vi "sendFixedData.vi"(8 "error in (no error)":errorcluster, 9 "File name wo extension":string="AdminConfig", 10 "File contents":string, 11 "SM1000-control in":T1) -> (0 "error out":errorcluster, 3 "SM1000-control out":T1)   [LabVIEW 2013, in "SLMControl.lvlib" / "SM1000.lvclass"]
doc: "Send fixed data to an EC device session.\n\nData retrieved via the 'requestFixedData' method may be modified and passed back to the controller for local storage. That data will then be immediately used and also the next time the module is booted.\nAn application should wait on an application message event 'FixedDataProcessed' to be assured the updated data has been processed by the EC1000 and is ready for subsequent actions."
uses:
  SM1000.lvclass
  Object-reference.ctl
  SM1000.lvclass/SM1000.ctl
  Custom-errors.ctl
  C:/Users/vangeste/Desktop/2015-06-02 - SLM - MAIF/HC-HardwareCharacterization/Sources/SM1000/LECSession.dll
  HC-HardwareCharacterization/Sources/SM1000/LECSession.dll
  DOTNET-error-int.vi
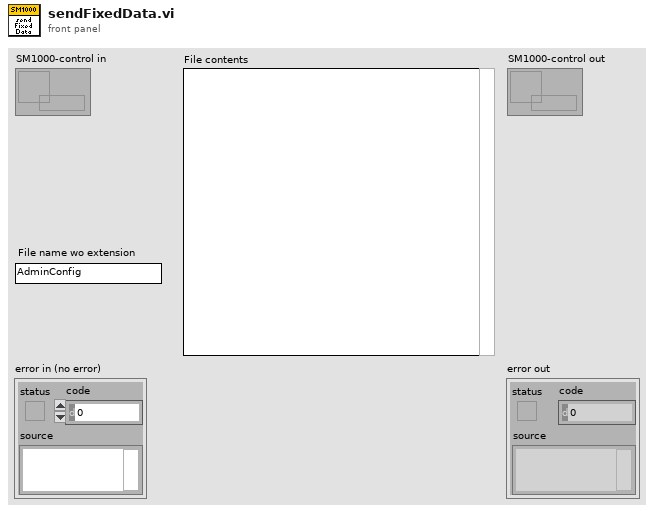
[diagram p1: front panel]
types:
  T1 = typedef "SLMControl.lvlib/SM1000.lvclass/Object-reference.ctl" = refnum<data-value>
  T2 = typedef "SLMControl.lvlib/SM1000.lvclass/Custom-errors.ctl" = enum16{"No error", "Not implemented", "Command not recognized", "Invalid input", "No connection", "Timeout", "Resource not loaded"}
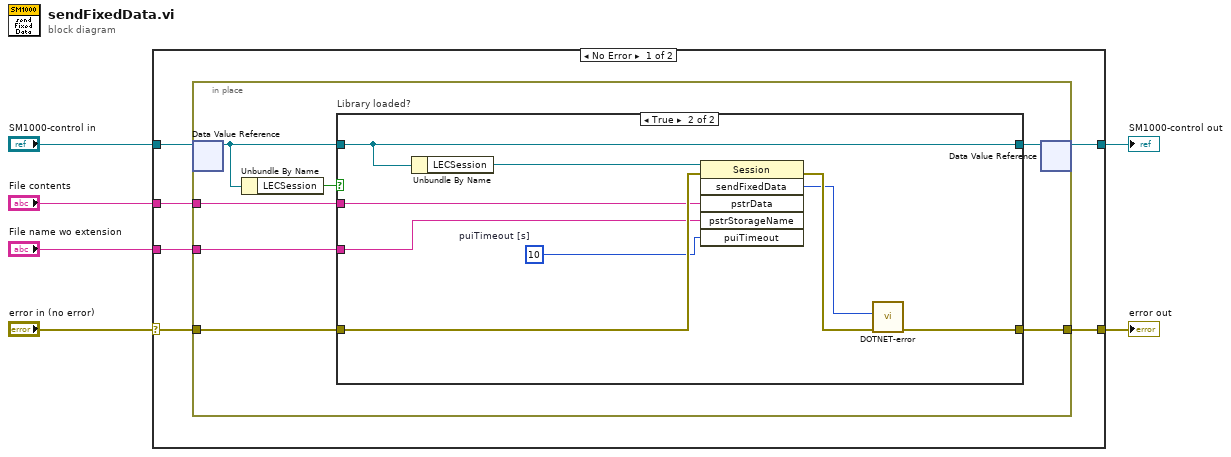
[diagram p0: block diagram]
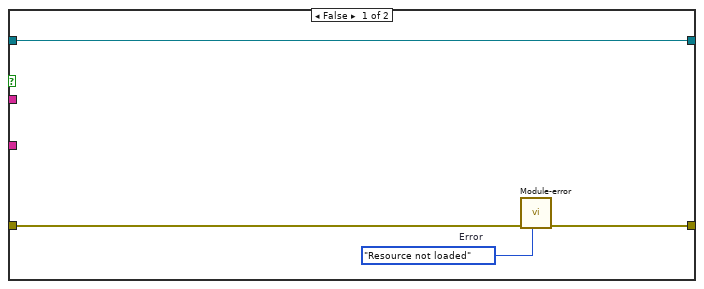
[diagram p2: hidden frame]
diagram:
  n1 = case shown="No Error" "error in (no error)" {
    selector: "error in (no error)" -> [w10 w34]
    tunnel: [w9 w34] -> w5
    tunnel: [w11 w33] -> w3
    tunnel: "SM1000-control in" -> [w12 w33]
    tunnel: "File name wo extension" -> [w8 _]
    tunnel: "File contents" -> [w7 _]
    frame No Error {
      n2 = in-place {
        in-place-border: w10 -> [w19]
        in-place-border: [w16] -> w9
        in-place-border: w8 -> [w14]
        in-place-border: w7 -> [w13]
        n3 = in-place-dvr #1(w12) -> (w17:refnum<class "SM1000.lvclass">)  [unwired: 1 out]
        n4 = Unbundle By Name(w17) -> ("LECSession"=w18:bool)
        n5 = case "Library loaded?" shown="True" w18 {
          tunnel: w19 -> [w23 w31]
          tunnel: w17 -> [w21 w29]
          tunnel: [w22 w26] -> w16
          tunnel: [w21 w29] -> w15
          tunnel: w14 -> [_ w30]
          tunnel: w13 -> [_ w28]
          frame False {
            w20 = Custom-errors."Resource not loaded"  # Error
            n6 = call "Module-error.vi"("Error"=w20, "error in (no error)"=w23) -> ("error out"=w22:errorcluster)  [unwired: 9 in]
          }
          frame True {
            w27 = u32 10  # puiTimeout [s]
            n7 = Unbundle By Name(w29) -> ("LECSession"=w32:refnum<k24>)
            n8 = invoke class="Session" method="sendFixedData"(reference=w32, error in=w31, "pstrData"=w28, "pstrStorageName"=w30, "puiTimeout"=w27) -> (error out=w25:errorcluster, "sendFixedData"=w24:u32)  [unwired: 1 in, 4 out]
            n9 = call-poly "DOTNET-error.vi"("error in (no error)"=w25, "Retun code"=w24) -> ("error out"=w26:errorcluster)  [unwired: 9 in]
          }
        }
        n10 = in-place-dvr #1(w15) -> (w11:T1)  [unwired: 1 out]
      }
    }
    frame Error {
    }
  }
  "error out" <- w5
  "SM1000-control out" <- w3
